vi "Script Interpreter(SubVI).vi"(8 "error in (no error)":errorcluster, 9 "Transd IN":u64[](array[numeric]), 10 "Data IN":string[](array[string]), 11 "Tamaño trama":u32) -> (0 "error out":errorcluster, 2 "Raw Data":T1, 3 "Checksum":bool)   [LabVIEW 2014, in "CAP-USB.lvlib"]
uses:
  CAP-USB.lvlib
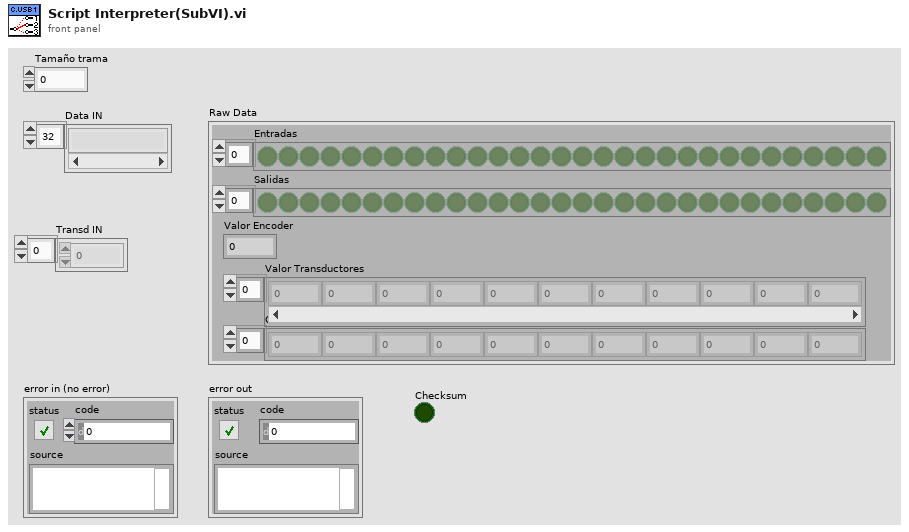
[diagram p1: front panel]
types:
  T1 = cluster{"Entradas":bool[], "Salidas":bool[], "Valor Encoder":u16, "Valor Transductores":u16[], "Orden Transd":i32[]}
  T2 = cluster{"Entradas":bool[], "Salidas":bool[], "VALOR ENCODER":u16, "Valor Transductores":u16[], "Transd IN":u64[]}
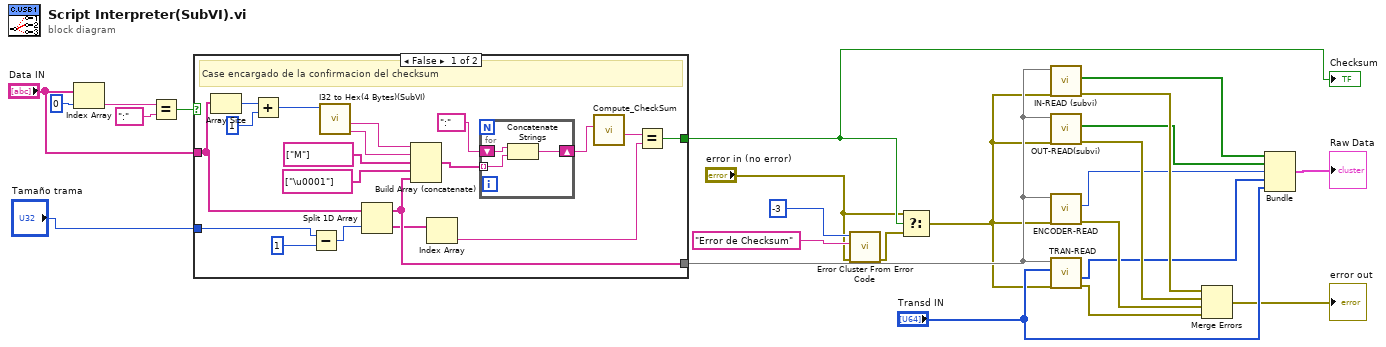
[diagram p0: block diagram]
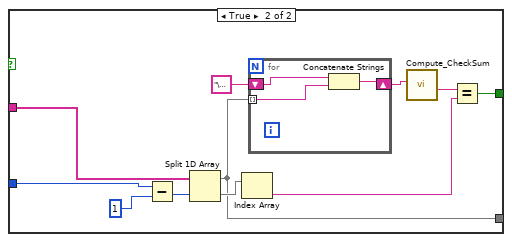
[diagram p2: hidden frame]
diagram:
  n1 = Index Array(array="Data IN", index=0) -> (element=w11:string)
  n2 = Equal?(x=w11, y=":") -> (x = y?=w9:bool)
  n3 = case shown="False" w9 {
    tunnel: [w43 w57] -> w3
    tunnel: "Tamaño trama" -> [w39 w56]
    tunnel: [w38 w49] -> w19
    tunnel: "Data IN" -> [w25 w50]
    frame False {
      # "Case encargado de la confirmacion del checksum"
      n4 = Array Size(array=w25) -> (size(s)=w36:i32)
      n5 = Add(x=w36, y=1) -> (x+y=w42:i32)
      n6 = Subtract(x=w39, y=u32 1) -> (x-y=w34:u32)
      n7 = call "I32 to Hex(4 Bytes)(SubVI).vi"("I32"=w42) -> ("BYTE 3"=w40:string, "BYTE 2"=w41:string)  [unwired: 6 in, 3 out]
      n8 = Split 1D Array(array=w25, index=w34) -> (first subarray=w38:string[], second subarray=w32:string[])
      n9 = Build Array (concatenate)(w41, w40, string[] ["M"] ("array"), string[] ["\u0001"] ("array"), w38) -> (w29:string[])
      n10 = Index Array(array=w32) -> (element=w33:string)  [unwired: 1 in]
      n11 = for {
        tunnel: w29 -> [w46] mode=indexing
        shift-right: [w45] -> w31
        shift-left: ":" -> [w44]
        n12 = Concatenate Strings(w44, w46) -> (w45:string)
      }
      n13 = call "Compute_CheckSum.vi"("Trama IN"=w31) -> ("Checksum ASCII"=w26:string)  [unwired: 9 in, 1 out]
      n14 = Equal?(x=w26, y=w33) -> (x = y?=w43:bool)
    }
    frame True {
      n15 = Subtract(x=w56, y=u32 1) -> (x-y=w54:u32)
      n16 = Split 1D Array(array=w50, index=w54) -> (first subarray=w49:string[], second subarray=w52:string[])
      n17 = Index Array(array=w52) -> (element=w53:string)  [unwired: 1 in]
      n18 = for {
        tunnel: w49 -> [w59] mode=indexing
        shift-right: [w60] -> w47
        shift-left: "\u0000" -> [w58]
        n19 = Concatenate Strings(w58, w59) -> (w60:string)
      }
      n20 = call "Compute_CheckSum.vi"("Trama IN"=w47) -> ("Checksum ASCII"=w51:string)  [unwired: 9 in, 1 out]
      n21 = Equal?(x=w51, y=w53) -> (x = y?=w57:bool)
    }
  }
  "Checksum" <- w3
  n22 = call <vilib>:"Error Cluster From Error Code.vi"("error in (no error)"="error in (no error)", "error message (\"\")"="Error de Checksum", "error code (0)"=-3) -> ("error out"=w1:errorcluster)  [unwired: 6 in]
  n23 = Select(t="error in (no error)", s=w3, f=w1) -> (s? t:f=w4:errorcluster)
  n24 = call "IN-READ (subvi).vi"("error in (no error)"=w4, "ARRAY IN"=w19) -> ("error out"=w20:errorcluster, "Entradas"=w15:bool[])  [unwired: 8 in]
  n25 = call "OUT-READ(subvi).vi"("error in (no error)"=w4, "ARRAY IN"=w19) -> ("error out"=w21:errorcluster, "Salidas"=w16:bool[])  [unwired: 8 in]
  n26 = call "ENCODER-READ.vi"("error in (no error)"=w4, "ARRAY IN"=w19) -> ("error out"=w22:errorcluster, "VALOR ENCODER"=w7:u16)  [unwired: 8 in]
  n27 = call "TRAN-READ.vi"("error in (no error)"=w4, "Numero de transd"="Transd IN", "ARRAY IN"=w19) -> ("error out"=w23:errorcluster, "Valor Transductores"=w17:u16[])  [unwired: 7 in]
  n28 = Merge Errors(w20, w21, w22, w23) -> (→"error out":errorcluster)
  n29 = Bundle("Entradas"=w15, "Salidas"=w16, "VALOR ENCODER"=w7, "Valor Transductores"=w17, "Transd IN"="Transd IN") -> (→"Raw Data":T2)  [unwired: 1 in]
